vi "ALTS-2015 Write PC ACK tag with delay.vi"(8 "error in (no error)":errorcluster, 11 "Tags Read?":i32) -> (0 "error out":errorcluster)   [LabVIEW 2013]
uses:
  Sub VIs/OPC Engine/Controls/ALTS-2015 OPC Write Registers.ctl
  Sub VIs/OPC Engine/Controls/ALTS-2015 OPC Write Global Options.ctl
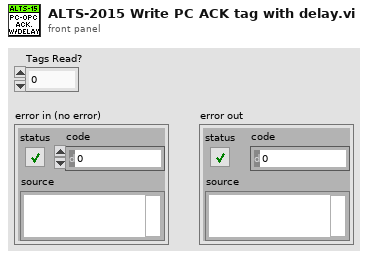
[diagram p1: front panel]
types:
  T1 = typedef "ALTS-2015 OPC Write Global Options.ctl" = enum16{"Init", "Write Value", "Write Array", "Read Value", "Read Array", "Read All"}
  T2 = typedef "ALTS-2015 OPC Write Registers.ctl" = enum16{"Task_Available_for_Robot", "New_Serial", "Serial_Adapter_Size", "Serial_Displacement_Size", "Serial_Flange_Size", "Test_Result", "Station_Number", "Rerun", "Invalid_SNo", "PC_ACK_Read_Tags"}
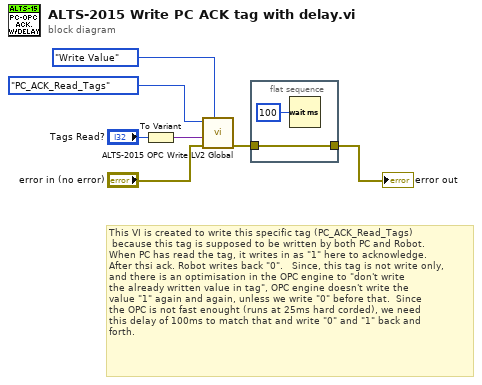
[diagram p0: block diagram]
diagram:
  # "This VI is created to write this specific tag (PC_ACK_Read_Tags)\n because this tag is supposed to be written by both PC and Robot.\nWhen PC has read the tag, it writes in as \"1\" here to acknowledge.\nAfter thsi ack. Robot writes back \"0\".   Since, this tag is not write only,\nand there is an optimisation in the OPC engine to \"don't write\nthe already written value in tag\", OPC engine doesn't write the \nvalue \"1\" again and again, unless we write \"0\" before that.  Since\nthe OPC is not fast enought (runs at 25ms hard corded), we need\nthis delay of 100ms to match that and write \"0\" and \"1\" back and\nforth."
  n1 = To Variant(anything="Tags Read?") -> (Variant=w5:variant)
  n2 = call "ALTS-2015 OPC Write LV2 Global.vi"("Options"=ALTS-2015_OPC_Write_Global_Options."Write Value", "error in (no error)"="error in (no error)", "OPC value"=w5, "OPC Write Register"=ALTS-2015_OPC_Write_Registers."PC_ACK_Read_Tags") -> ("error out"=w1:errorcluster)  [unwired: 5 in, 2 out]
  n3 = flat-sequence {
    tunnel: [w8] -> w2
    tunnel: w1 -> [w8]
    frame #0 {
      n4 = Wait (ms)(milliseconds to wait=u32 100) -> ()  [unwired: 1 out]
    }
  }
  "error out" <- w2
